vi "EQE_MoveToWavelength.vi"(0 "Input Wavelength":dbl) -> (1 "Error Code":i32, 2 "Current Wavelength":dbl)   [LabVIEW 2017]
uses:
  Program Files (x86)/Bentham/SDK/code examples/LabView/8.0/BenHw/benhw32_stdcall.dll
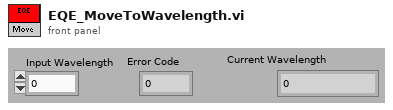
[diagram p1: front panel]
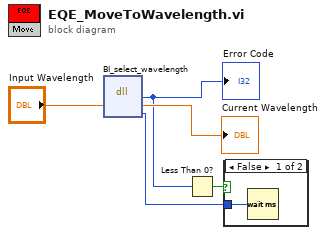
[diagram p0: block diagram]
diagram:
  n1 = dll-call lib="C:/Program Files (x86)/Bentham/SDK/code examples/LabView/8.0/BenHw/benhw32_stdcall.dll" fn="BI_select_wavelength"("wl"="Input Wavelength") -> (w1:i16, "wl"=→"Current Wavelength":dbl, "settle_delay"=w2:i32)  [unwired: 4 in, 2 out]
  "Error Code" <- w1
  n2 = Less Than 0?(x=w1) -> (x < 0?=w3:bool)
  n3 = case shown="False" w3 {
    tunnel: w2 -> [w6 _]
    frame False {
      n4 = Wait (ms)(milliseconds to wait=w6) -> ()  [unwired: 1 out]
    }
    frame True {
    }
  }
